vi "Read extensions.vi"(11 "connection in":refnum<class "Low Level Connection.lvclass">) -> (2 "extensions":set{T1}(c389), 3 "connection out":refnum<class "Low Level Connection.lvclass">)   [LabVIEW 2020, in "NI_SFTP.lvlib" / "Low Level Connection.lvclass"]
uses:
  <vilib>/net/SFTP/Low Level Connection/Low Level Connection.lvclass
  <vilib>/net/SFTP/Low Level Connection/Extension Pair.ctl
  <vilib>/net/SFTP/Low Level Connection/Low Level Connection.lvclass/Low Level Connection.ctl
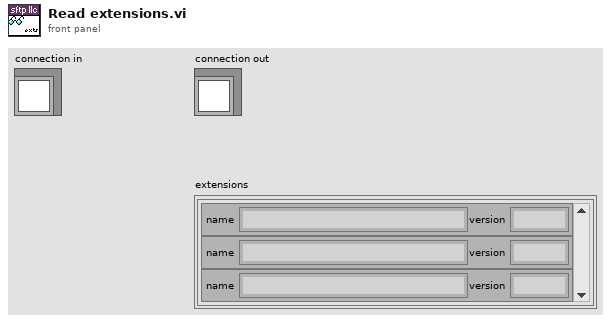
[diagram p1: front panel]
types:
  T1 = typedef "NI_SFTP.lvlib/Low Level Connection.lvclass/Extension Pair.ctl" = cluster{"name":string, "version":string}
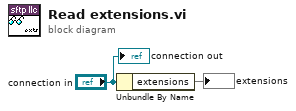
[diagram p0: block diagram]
diagram:
  n1 = Unbundle By Name("connection in") -> ("extensions"=→"extensions":set{cluster{"name":string, "version":string}})
  "connection out" <- "connection in"
